vi "NI VeriStand - Get Item GUID.vi"(8 "error in (no error)":errorcluster, 11 "Item Ref in":T1 format="%.0x") -> (0 "error out":errorcluster, 2 "GUID":string, 3 "Item Ref out":T1 format="%.0x")   [LabVIEW 2020, in "Custom Device API.lvlib"]
doc: "Returns the <B>GUID</B> of the configuration page associated with a custom device item, as defined in the custom device XML file."
uses:
  <vilib>/NI VeriStand/Custom Device API/Custom Device API.lvlib
  <vilib>/NI VeriStand/Custom Device API/Custom Device Item Ref.ctl
  5479ba10-a2b3-4fa3-a26e-96cdf2ba7dc7.vi
  <vilib>/NI VeriStand/Custom Device API/Custom Device Offline Path.vi
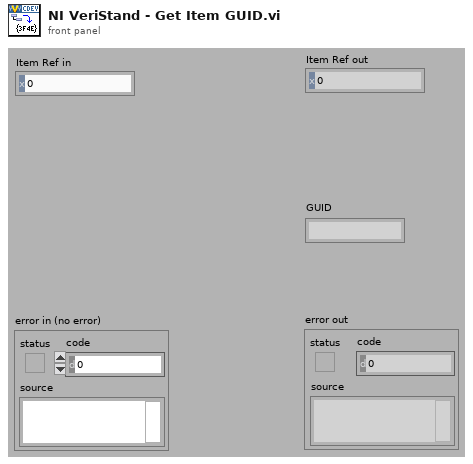
[diagram p1: front panel]
types:
  T1 = typedef "Custom Device API.lvlib/Custom Device Item Ref.ctl" = u64
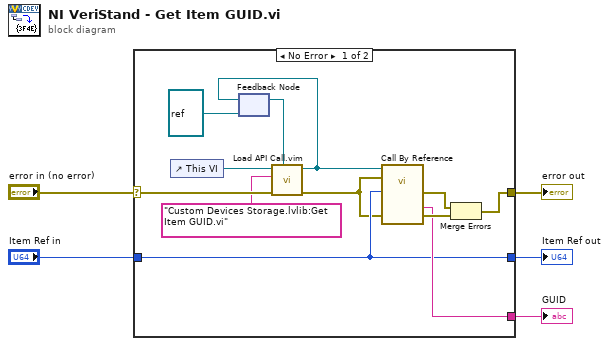
[diagram p0: block diagram]
diagram:
  n1 = case shown="No Error" "error in (no error)" {
    selector: "error in (no error)" -> [w11 w19]
    tunnel: [w16 w19] -> w5
    tunnel: "Item Ref in" -> [w14 w18]
    tunnel: [w14 w18] -> w3
    tunnel: [w15 _] -> w2
    frame No Error {
      n2 = control-ref of="This VI"() -> (w12:refnum<vi>)
      n3 = feedback #1(refnum<vi> refnum ("type specifier VI Refnum (for type only)")) -> (w13:refnum<vi>)
      n4 = call "Load API Call.vim"("VI reference in"=w13, "error in (no error)"=w11, "VI qualified name"="Custom Devices Storage.lvlib:Get Item GUID.vi", "Caller VI ref"=w12) -> ("error out"=w10:errorcluster, "VI reference"=w9:refnum<vi>)  [unwired: 6 in]
      n5 = feedback-in #1(w9) -> ()
      n6 = call-by-ref "?"(reference=w9, error in=w10, 8:"error in (no error)"=w10, "Item Ref in"=w14) -> (error out=w6:errorcluster, 0:"error out"=w17:errorcluster, "GUID"=w15:string)  [unwired: 7 in, 2 out]
      n7 = Merge Errors(w6, w17) -> (w16:errorcluster)
    }
    frame Error {
    }
  }
  "error out" <- w5
  "Item Ref out" <- w3
  "GUID" <- w2
